vi "MenuConfig_ColorWrite.vi"(8 "error in (no error)":errorcluster, 9 "Colors[4]":cluster{u32, u32}[](array[cluster]), 10 "Color.Name (\"Default\")":string="Default", 11 "MenuConfig":variant) -> (0 "error out":errorcluster, 3 "MenuConfig":variant)   [LabVIEW 2019, in "Menu Button.xctl"]
doc: "JSMA Module Template - Top Level UI 0.2.0.4\nRob Humfeld - Jet Engineering\nCopyright (c) 2019, Jet Engineering"
uses:
  Menu Button.xctl
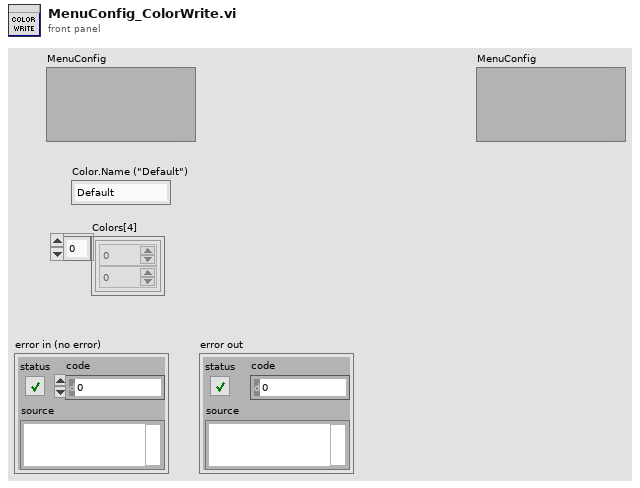
[diagram p1: front panel]
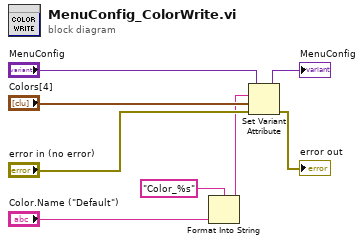
[diagram p0: block diagram]
diagram:
  n1 = Format Into String(format string="Color_%s" ("name"), "Color.Name (\"Default\")") -> (resulting string=w3:string)  [unwired: 2 in, 1 out]
  n2 = Set Variant Attribute(Variant="MenuConfig", name=w3, value="Colors[4]", error in="error in (no error)") -> (Variant out=→"MenuConfig":variant, error out=→"error out":errorcluster)  [unwired: 1 out]
